vi "CreateMaskFromROI.vi"(8 "error in (no error)":errorcluster, 10 "Settings":T1={"Harware Configuration"={"Camera"="cam1", "Frames Per Second"=15, "Simulate Recording"=FALSE, "Simulated Recording Sample"=path "", "Timestamp Method"=enum."Camera Timestamp"}, "Base Recording Path"=path "", "Type Of Recording"="", "Recording Codec"="", "TrackingSettings"={"Max Radius"=0, "Threshold"=160.0, "ROI"={"Left"=0, "Top"=0, "Right"=0, "Bottom"=0, "Rotation"=0.0}}, "Calibration"={"Pixel Width (X)"=10.0, "Pixel Height (Y)"=100.0}, "Broadcast Length"=0} {"Broadcast Length" min=0; "TrackingSettings"."ROI"."Rotation" format="%.2f"; "TrackingSettings"."ROI"."Left" scale=0.0..1024.0; "TrackingSettings"."ROI"."Right" scale=0.0..1024.0; "TrackingSettings"."Threshold" scale=0.0..255.0}, 11 "?":T6) -> (0 "error out":errorcluster, 2 "Settings 2":T1={"Harware Configuration"={"Camera"="cam1", "Frames Per Second"=15, "Simulate Recording"=FALSE, "Simulated Recording Sample"=path "", "Timestamp Method"=enum."Camera Timestamp"}, "Base Recording Path"=path "", "Type Of Recording"="", "Recording Codec"="", "TrackingSettings"={"Max Radius"=0, "Threshold"=160.0, "ROI"={"Left"=0, "Top"=0, "Right"=0, "Bottom"=0, "Rotation"=0.0}}, "Calibration"={"Pixel Width (X)"=10.0, "Pixel Height (Y)"=100.0}, "Broadcast Length"=0} {"Broadcast Length" min=0; "TrackingSettings"."ROI"."Rotation" format="%.2f"; "TrackingSettings"."ROI"."Left" scale=0.0..1024.0; "TrackingSettings"."ROI"."Right" scale=0.0..1024.0; "TrackingSettings"."Threshold" scale=0.0..255.0}, 3 "output cluster":T6)   [LabVIEW 2017, in "ImageAcquisitionLibrary.lvlib"]
uses:
  ImageAcquisitionLibrary.lvlib
  TrackingImages.ctl
  <vilib>/vision/Image Controls.llb/IMAQ Image.ctl
  Settings/Settings.ctl
  <vilib>/userdefined/High Color/IMAQdx.ctl
  Tracking/TrackingSettings.ctl
  Settings/Calibration.ctl
  <vilib>/vision/NI_Vision_Development_Module.lvlib
panel:
  out "Coordinates out of space?":bool
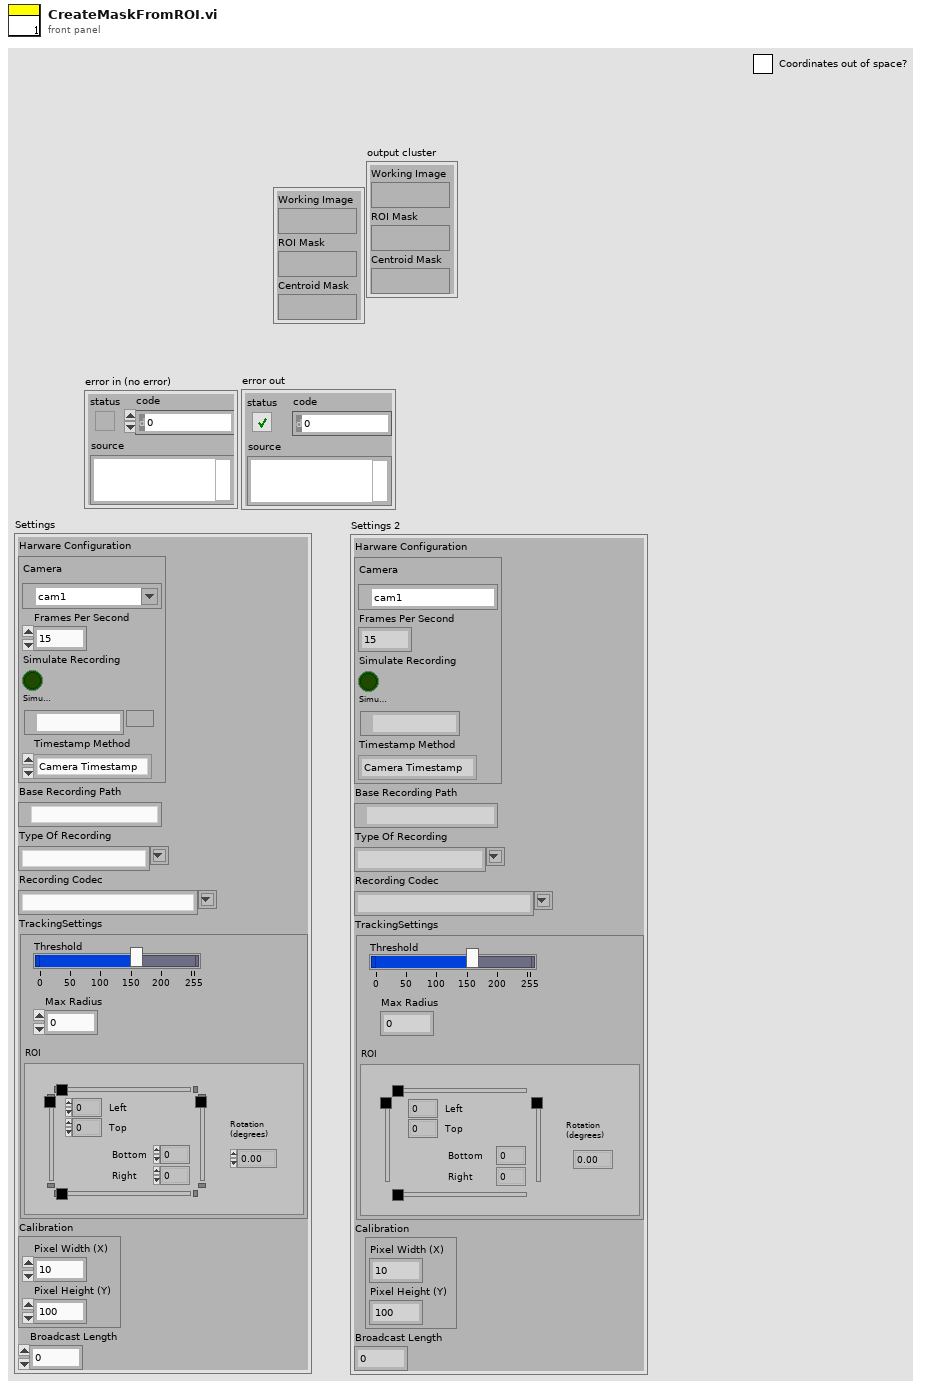
[diagram p1: front panel]
types:
  T1 = typedef "ImageAcquisitionLibrary.lvlib/Settings.ctl" = cluster{"Harware Configuration":cluster{"Camera":T2, "Frames Per Second":u32, "Simulate Recording":bool, "Simulated Recording Sample":path, "Timestamp Method":enum16{"System Timestamp", "Camera Timestamp", "IMAQdx Timestamp"}}, "Base Recording Path":path, "Type Of Recording":string, "Recording Codec":string, "TrackingSettings":T3, "Calibration":T5, "Broadcast Length":i32}
  T2 = typedef "IMAQdx.ctl" = refnum<k21>
  T3 = typedef "ImageAcquisitionLibrary.lvlib/TrackingSettings.ctl" = cluster{"Max Radius":i32, "Threshold":sgl, "ROI":T4}
  T4 = typedef "IMAQ Rectangle" = cluster{"Left":i32, "Top":i32, "Right":i32, "Bottom":i32, "Rotation":dbl}
  T5 = typedef "ImageAcquisitionLibrary.lvlib/Calibration.ctl" = cluster{"Pixel Width (X)":dbl, "Pixel Height (Y)":dbl}
  T6 = typedef "ImageAcquisitionLibrary.lvlib/TrackingImages.ctl" = cluster{"Working Image":T7, "ROI Mask":T7, "Centroid Mask":T7}
  T7 = typedef "IMAQ Image.ctl" = refnum<image>
  T8 = typedef "ROI Descriptor" = cluster{"Global Rectangle":i32[], "Contours":cluster{"ID":enum32{"External", "Internal"}, "Type":u32, "Coordinates":i32[]}[]}
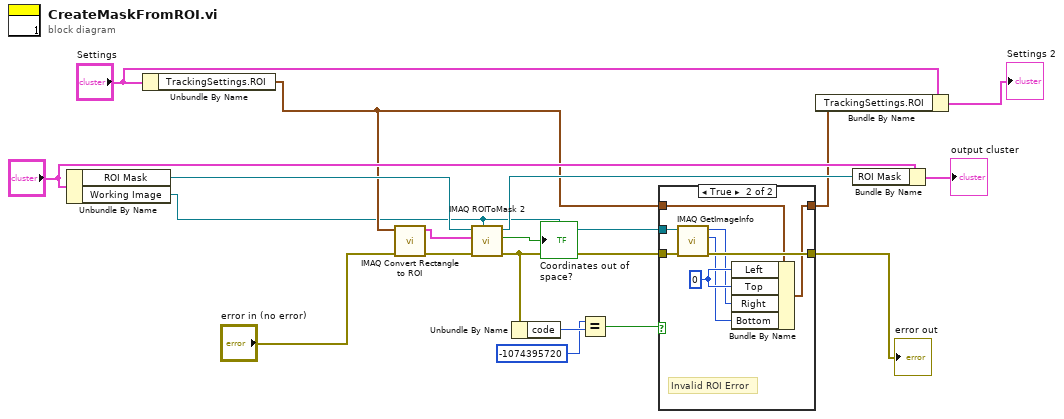
[diagram p0: block diagram]
diagram:
  n1 = Unbundle By Name("?") -> ("ROI Mask"=w15:T7, "Working Image"=w6:T7)
  n2 = Unbundle By Name("Settings") -> ("TrackingSettings.ROI"=w10:T4)
  n3 = call "IMAQ Convert Rectangle to ROI"("error in (no error)"="error in (no error)", "Rectangle"=w10) -> ("error out"=w17:errorcluster, "ROI Descriptor"=w18:T8)  [unwired: 7 in]
  n4 = call "IMAQ ROIToMask 2"("Image Model"=w6, "error in (no error)"=w17, "ROI Descriptor"=w18, "Image"=w15) -> ("error out"=w5:errorcluster, "Coordinates out of space?"=→"Coordinates out of space?":bool, "Image Out"=w11:T7)  [unwired: 5 in]
  n5 = Unbundle By Name(w5) -> ("code"=w4:i32)
  n6 = Equal?(x=-1074395720 ("code"), y=w4) -> (x = y?=w3:bool)
  n7 = case shown="True" w3 {
    tunnel: [w20 w27] -> w12
    tunnel: w5 -> [w20 w28]
    tunnel: w6 -> [_ w26]
    tunnel: w10 -> [w19 w25]
    tunnel: [w19 w21] -> w8
    frame False {
    }
    frame True {
      w24 = 0 ("Left")
      # "Invalid ROI Error"
      n8 = call "IMAQ GetImageInfo"("error in (no error)"=w28, "Image"=w26) -> ("error out"=w27:errorcluster, "Y Resolution"=w23:i32, "X Resolution"=w22:i32)  [unwired: 2 in, 5 out]
      n9 = Bundle By Name(cluster=w25, "Left"=w24, "Top"=w24, "Right"=w22, "Bottom"=w23) -> (w21:T4)
    }
  }
  "error out" <- w12
  n10 = Bundle By Name(cluster="Settings", "TrackingSettings.ROI"=w8) -> (→"Settings 2":T1)
  n11 = Bundle By Name(cluster="?", "ROI Mask"=w11) -> (→"output cluster":T6)
